vi "ARC_Queue Insert Element.vi"(6 "at front (F)":bool caption="At Front? (F)", 7 "Time out(-1)_queue in":i32=-1 caption="Time Out(-1)_Queue In", 8 "error in (no error)":errorcluster caption="Error In (no error)", 9 "Data":variant, 10 "Event":string, 11 "Queue Name(unamed)":string) -> (0 "error out":errorcluster caption="Error Out", 2 "Timed Out?":bool)   [LabVIEW 2016]
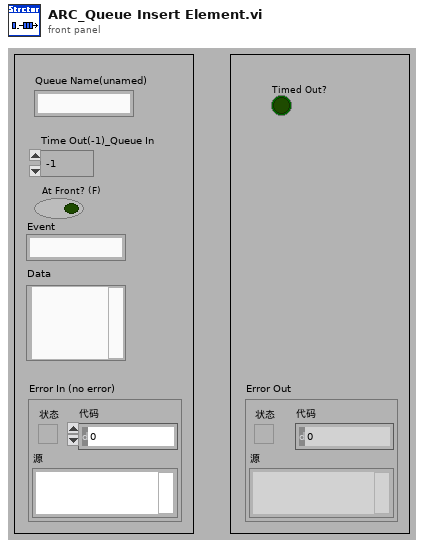
[diagram p1: front panel]
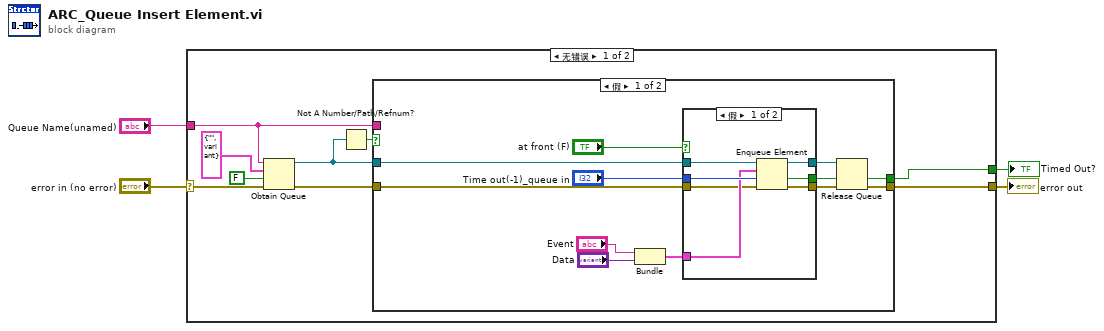
[diagram p0: block diagram]
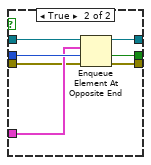
[diagram p2: hidden frame]
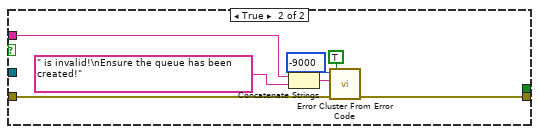
[diagram p3: hidden frame]
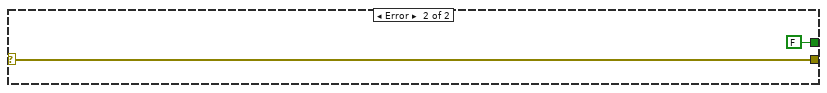
[diagram p4: hidden frame]
diagram:
  n1 = case shown="无错误" "error in (no error)" {
    selector: "error in (no error)" -> [w8 w47]
    tunnel: [w13 w47] -> w3
    tunnel: "Queue Name(unamed)" -> [w7 _]
    tunnel: [w6 FALSE ("timed out?")] -> w1
    frame No Error {
      n2 = Obtain Queue(name (unnamed)=w7, element data type=cluster{"Event":string, "Data":variant} {"Event"="", "Data"=variant} ("输出簇"), create if not found? (T)=FALSE ("如未找到是否创建？(T)"), error in (no error)=w8) -> (queue out=w10:refnum<queue>, error out=w12:errorcluster)  [unwired: 1 in, 1 out]
      n3 = Not A Number/Path/Refnum?(number/path/refnum=w10) -> (NaN/Path/Refnum?=w9:bool)
      n4 = case shown="假" w9 {
        tunnel: w12 -> [w21 w40]
        tunnel: [w15 w39] -> w13
        tunnel: w7 -> [_ w41]
        tunnel: [w20 _] -> w6
        tunnel: w10 -> [w19 _]
        frame False {
          n5 = Bundle("Event"="Event", "Data"="Data") -> (w14:cluster{"Event":string, "Data":variant})  [unwired: 1 in]
          n6 = case shown="假" "at front (F)" {
            tunnel: "Time out(-1)_queue in" -> [w31 w37]
            tunnel: w14 -> [w30 w36]
            tunnel: w21 -> [w29 w35]
            tunnel: [w28 w34] -> w17
            tunnel: [w27 w33] -> w20
            tunnel: w19 -> [w26 w38]
            tunnel: [w25 w32] -> w16
            frame False {
              n7 = Enqueue Element(queue=w26, element=w30, timeout in ms (-1)=w31, error in (no error)=w29) -> (queue out=w25:refnum<queue>, timed out?=w27:bool, error out=w28:errorcluster)
            }
            frame True {
              n8 = Enqueue Element At Opposite End(queue=w38, element=w36, timeout in ms (-1)=w37, error in (no error)=w35) -> (queue out=w32:refnum<queue>, timed out?=w33:bool, error out=w34:errorcluster)
            }
          }
          n9 = Release Queue(queue=w16, error in (no error)=w17) -> (error out=w15:errorcluster)  [unwired: 1 in, 2 out]
        }
        frame True {
          n10 = Concatenate Strings(w41, " is invalid!\nEnsure the queue has been created!" ("字符串")) -> (w43:string)
          n11 = call <vilib>:"Error Cluster From Error Code.vi"("show call chain? (False)"=TRUE, "error in (no error)"=w40, "error message (\"\")"=w43, "error code (0)"=-9000) -> ("error out"=w39:errorcluster)  [unwired: 5 in]
        }
      }
    }
    frame Error {
    }
  }
  "error out" <- w3
  "Timed Out?" <- w1
